vi "CALC_EQU_TEXT.vi"(0 "VISA IN":refnum<visa-resource-name>, 1 "Equation or Expression":string, 5 "error in":errorcluster, 7 "Channel":i32) -> (14 "VISA Out":refnum<visa-resource-name>, 19 "error out":errorcluster)   [LabVIEW 2018, in "PNA-X.lvlib"]
doc: "CALCulate<cnum>:EQUation:TEXT <string> \n(Read-Write) Specifies an equation or expression to be used on the selected measurement for the \nspecified channel. \nSee Critical Note \nParameters \n<cnum> Channel number of the measurement. There must be a selected measurement \non that channel. If unspecified, <cnum> is set to 1. \n<string> Any valid equation or expression. See Equation Editor. \nExamples 'Equation (includes '=') \nCALC:EQU:TEXT \"foo=S11/S21\" \n'Expression \ncalculate2:equation:text \"S11/S21\" \nQuery Syntax CALCulate<cnum>:EQUation:TEXT? \nReturn Type String \nDefault Not Applicable"
uses:
  PNA-X.lvlib
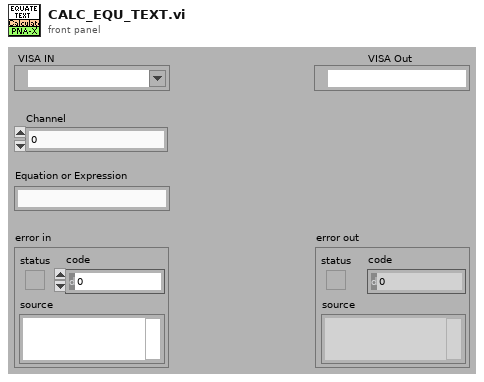
[diagram p1: front panel]
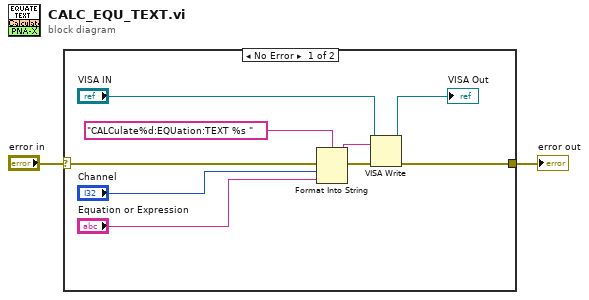
[diagram p0: block diagram]
diagram:
  n1 = case shown="No Error" "error in" {
    selector: "error in" -> [w11 w12]
    tunnel: [w6 w12] -> w1
    frame No Error {
      n2 = Format Into String(format string="CALCulate%d:EQUation:TEXT %s " ("Cmdline"), error in=w11, "Channel", "Equation or Expression") -> (resulting string=w9:string, error out=w10:errorcluster)  [unwired: 1 in]
      n3 = VISA Write(VISA resource name="VISA IN", write buffer=w9, error in (no error)=w10) -> (VISA resource name out=→"VISA Out":refnum<visa-resource-name>, error out=w6:errorcluster)  [unwired: 1 out]
    }
    frame Error {
    }
  }
  "error out" <- w1
